vi "StopGlobal.vi"() -> ()   [LabVIEW 2014, in "Nav6.lvlib"]
uses:
  Nav6.lvlib
panel:
  in  "Stop":bool
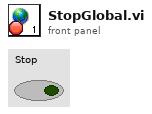
[diagram p1: front panel]
diagram:
